vi "Close.vi"(8 "error in":errorcluster, 11 "Synnax Client in":refnum<class "Synnax Client.lvclass">) -> (0 "error out":errorcluster, 3 "Synnax Client out":refnum<class "Synnax Client.lvclass">)   [LabVIEW 2026, in "synnax_clib.lvlib" / "Synnax Client.lvclass"]
uses:
  Synnax Client.lvclass
  Synnax Client.lvclass/Synnax Client.ctl
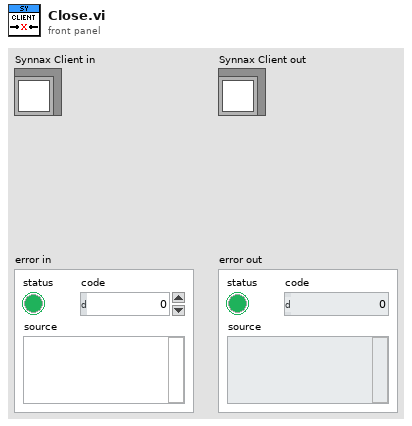
[diagram p1: front panel]
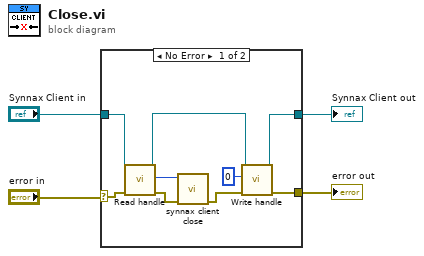
[diagram p0: block diagram]
diagram:
  n1 = case shown="No Error" "error in" {
    selector: "error in" -> [w8 w15]
    tunnel: [w13 w14] -> w1
    tunnel: [w12 w15] -> w2
    tunnel: "Synnax Client in" -> [w10 w14]
    frame No Error {
      n2 = call "Read handle.vi"("error in (no error)"=w8, "Synnax Client in"=w10) -> ("error out"=w7:errorcluster, "handle"=w11:u64, "Synnax Client out"=w9:refnum<class "Synnax Client.lvclass">)  [unwired: 7 in]
      n3 = call "synnax client close.vi"("error in"=w7, "client"=w11) -> ("error out"=w6:errorcluster)  [unwired: 9 in]
      n4 = call "Write handle.vi"("error in (no error)"=w6, "handle"=u64 0, "Synnax Client in"=w9) -> ("error out"=w12:errorcluster, "Synnax Client out"=w13:refnum<class "Synnax Client.lvclass">)  [unwired: 7 in]
    }
    frame Error {
    }
  }
  "error out" <- w2
  "Synnax Client out" <- w1
